vi "New.vi"(8 "error in (no error)":errorcluster, 11 "reference in":refnum<class "TemplateTestSuite.lvclass">) -> (0 "error out":errorcluster, 3 "reference out":refnum<class "TemplateTestSuite.lvclass">)   [LabVIEW 2013, in "TemplateTestSuite.lvclass"]
uses:
  TemplateTestSuite.lvclass
  Classes/TestCase/TestCase.lvclass
  TemplateTestSuite.lvclass/TemplateTestSuite.ctl
  Classes/TestSuite/TestSuite.lvclass
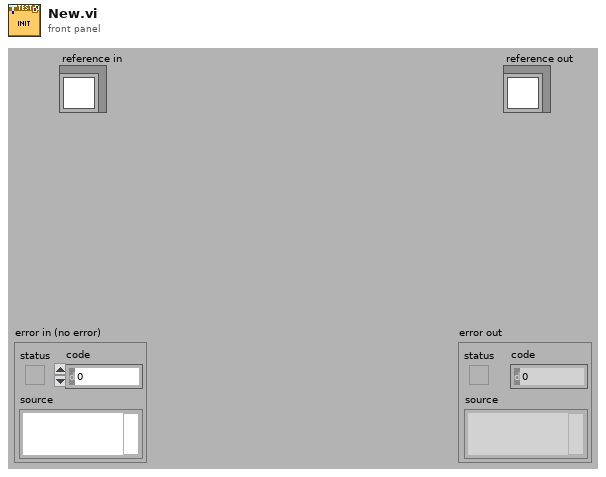
[diagram p1: front panel]
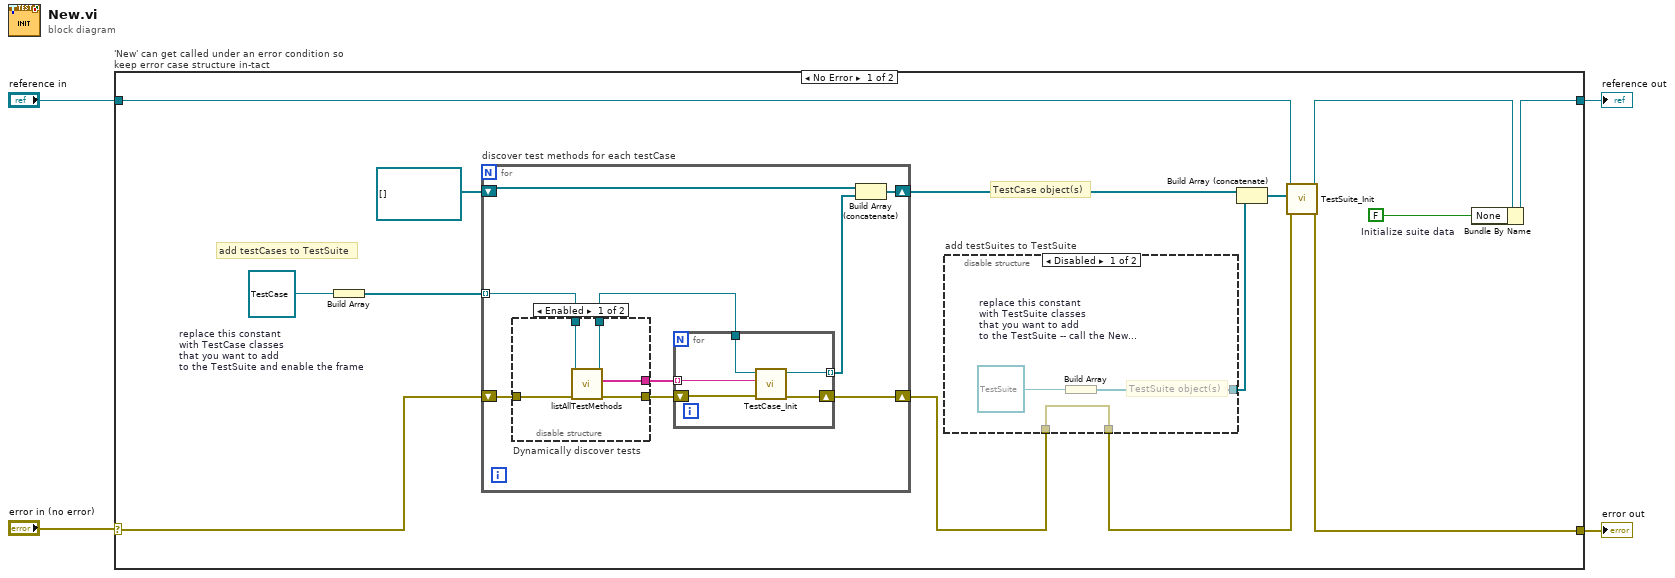
[diagram p0: block diagram]
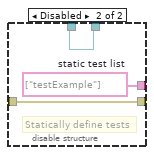
[diagram p2: hidden frame]
diagram:
  n1 = case "'New' can get called under an error condition so keep error case structure in-tact" shown="No Error" "error in (no error)" {
    selector: "error in (no error)" -> [w12 w45]
    tunnel: [w18 w46] -> w4
    tunnel: "reference in" -> [w13 w46]
    tunnel: [w15 w45] -> w1
    frame No Error {
      w6 = refnum<class "TestCase.lvclass"> refnum  # replace this constant with TestCase classes that you want to add to the TestSuite and enable the frame
      w17 = FALSE  # Initialize suite data
      # "TestCase object(s)"
      # "add testCases to TestSuite"
      n2 = Build Array(w6) -> (w14:refnum<class "TestCase.lvclass">[])
      n3 = for "discover test methods for each testCase" {
        shift-right: [w27] -> w7
        shift-left: w12 -> [w23]
        tunnel: w14 -> [w20] mode=indexing
        shift-right: [w24] -> w11
        shift-left: refnum<class "TestCase.lvclass">[] [] -> [w25]
        n4 = disable-structure "Dynamically discover tests" shown="Enabled" {
          disable-tunnel: w23 -> [w32 w33]
          disable-tunnel: [w31 w33] -> w22
          disable-tunnel: [w30 w34] -> w21
          disable-tunnel: w20 -> [w29 w35]
          disable-tunnel: [w28 w35] -> w19
          frame Enabled {
            n5 = call-dynamic "listAllTestMethods.vi"("error in (no error)"=w32, "TestCase in"=w29) -> ("error out"=w31:errorcluster, "test methods"=w30:string[], "TestCase out"=w28:refnum<class "TestCase.lvclass">)  [unwired: 7 in]
          }
          frame Disabled {
            w34 = string[] ["testExample"]  # static test list
            # "Statically define tests"
          }
        }
        n6 = for {
          tunnel: w19 -> [w36]
          tunnel: w21 -> [w40] mode=indexing
          shift-right: [w38] -> w27
          shift-left: w22 -> [w39]
          tunnel: [w37] -> w26 mode=indexing
          n7 = call "TestCase_Init.vi"("error in (no error)"=w39, "methodName (\"runTest\")"=w40, "TestCase in"=w36) -> ("error out"=w38:errorcluster, "TestCase out"=w37:refnum<class "TestCase.lvclass">)  [unwired: 7 in]
        }
        n8 = Build Array (concatenate)(w25, w26) -> (w24:refnum<class "TestCase.lvclass">[])
      }
      n9 = disable-structure "add testSuites to TestSuite" shown="Disabled" {
        disable-tunnel: [w41 _] -> w9
        disable-tunnel: [w43 w44] -> w8
        disable-tunnel: w7 -> [w43 w44]
        frame Disabled {
          w42 = refnum<class "TestSuite.lvclass"> refnum  # replace this constant with TestSuite classes that you want to add to the TestSuite -- call the New method for each TestSuite prior to adding it to this TestSuite
          # "TestSuite object(s)"
          n10 = Build Array(w42) -> (w41:refnum<class "TestSuite.lvclass">[])
        }
        frame Enabled {
          # "by default, no TestSuites are defined\nas members of a TestSuite"
        }
      }
      n11 = Build Array (concatenate)(w11, w9) -> (w10:refnum<class>[])
      n12 = call "TestSuite_Init.vi"("error in (no error)"=w8, "tests (none)"=w10, "TestSuite in"=w13) -> ("error out"=w15:errorcluster, "TestSuite out"=w16:refnum<class "TemplateTestSuite.lvclass">)  [unwired: 7 in]
      n13 = Bundle By Name(cluster=w16, "None"=w17) -> (w18:refnum<class "TemplateTestSuite.lvclass">)
    }
    frame Error {
    }
  }
  "reference out" <- w4
  "error out" <- w1
